vi "Write Swerve Speed Global.vi"(0 "Swerve 4":dbl, 1 "Swerve 3":dbl, 2 "Swerve 2":dbl, 3 "Swerve 1":dbl) -> ()   [LabVIEW 2016]
uses:
  Main/Robot Global Data.vi
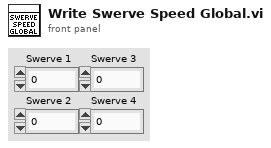
[diagram p1: front panel]
types:
  T1 = cluster{"Swerve 1":dbl, "Swerve 2":dbl, "Swerve 3":dbl, "Swerve 4":dbl}
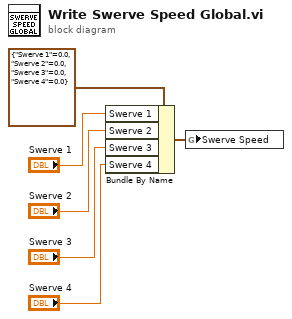
[diagram p0: block diagram]
diagram:
  n1 = Bundle By Name(cluster=T1 {"Swerve 1"=0.0, "Swerve 2"=0.0, "Swerve 3"=0.0, "Swerve 4"=0.0} ("input cluster"), "Swerve 1"="Swerve 1", "Swerve 2"="Swerve 2", "Swerve 3"="Swerve 3", "Swerve 4"="Swerve 4") -> (w6:T1)
  n2 = global write "Robot Global Data.vi" "Swerve Speed"(w6) -> ()
